vi "different random number.vi"(1 "New one":i32, 2 "Last one":i32, 3 "Max":i32) -> (0 "Final output":i32)   [LabVIEW 2016]
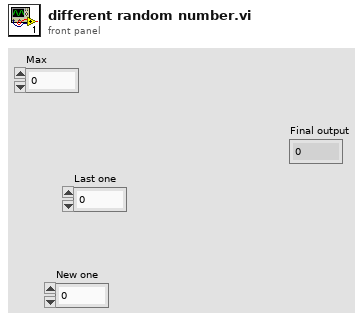
[diagram p1: front panel]
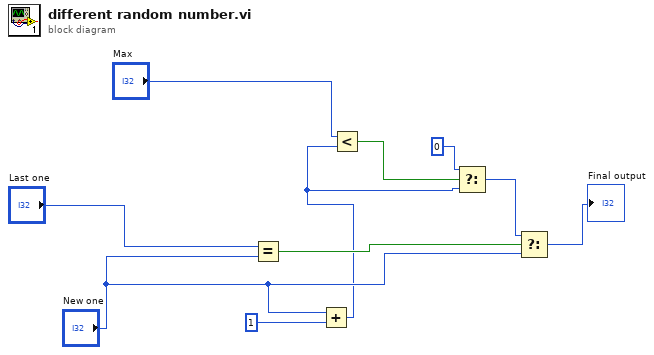
[diagram p0: block diagram]
diagram:
  n1 = Equal?(x="Last one", y="New one") -> (x = y?=w9:bool)
  n2 = Add(x="New one", y=1) -> (x+y=w3:i32)
  n3 = Less?(x="Max", y=w3) -> (x < y?=w5:bool)
  n4 = Select(t=0, s=w5, f=w3) -> (s? t:f=w2:i32)
  n5 = Select(t=w2, s=w9, f="New one") -> (s? t:f=→"Final output":i32)
